vi "Result.vi"(8 "error in (no error)":errorcluster, 10 "Result":T1={"Name"="", "Description"="", "Status"=enum."Passed", "Result Type"=enum."Test Suite", "Execution Time"=0.0, "Data"={"Expected"=variant, "Actual"=variant, "Delta"=variant}}, 11 "Execution Profiler In":refnum<class "Execution Profiler.lvclass">) -> (0 "error out":errorcluster, 3 "Execution Profiler Out":refnum<class "Execution Profiler.lvclass">)   [LabVIEW 2020, in "Execution Profiler.lvclass"]
uses:
  Execution Profiler.lvclass
  Core/Result/Result.ctl
  Core/Result/Status.ctl
  Core/Result/Type.ctl
  Execution Profiler.lvclass/Execution Profiler.ctl
  <vilib>/Utility/miscctls.llb/LVMapReplaceAction.ctl
  Core/Result/Result.lvlib
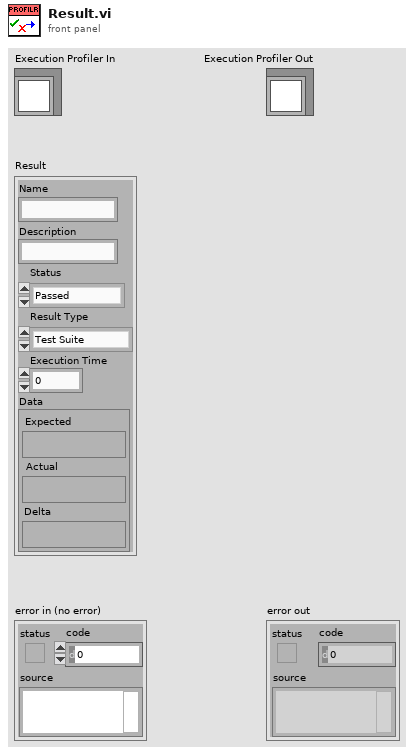
[diagram p1: front panel]
types:
  T1 = typedef "Result.lvlib/Result.ctl" = cluster{"Name":string, "Description":string, "Status":T2, "Result Type":T3, "Execution Time":dbl, "Data":cluster{"Expected":variant, "Actual":variant, "Delta":variant}}
  T2 = typedef "Result.lvlib/Status.ctl" = enum16{"", "Passed", "Failed", "Error", "Skipped", "Setup Error", "Broken", "Teardown Error"}
  T3 = typedef "Result.lvlib/Type.ctl" = enum16{"Test Case", "Test Suite", "Test Run", "Pass", "Fail", "Skip", "Pass if", "Fail if", "Pass if Error", "Fail if Error", "Pass if Equal", "Fail if Equal"}
  T4 = typedef "LVMapReplaceAction.ctl" = enum32{"Modify Entry only if found", "Add or Modify Entry", "Delete Entry"}
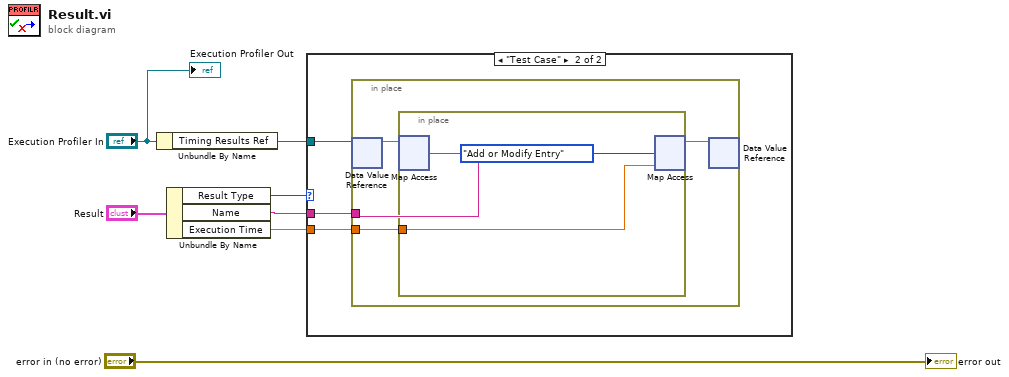
[diagram p0: block diagram]
diagram:
  n1 = Unbundle By Name("Execution Profiler In") -> ("Timing Results Ref"=w5:refnum<data-value>)
  n2 = Unbundle By Name("Result") -> ("Result Type"=w1:T3, "Name"=w4:string, "Execution Time"=w2:dbl)
  n3 = case shown="\"Test Case\"" w1 {
    tunnel: w5 -> [_ w10]
    tunnel: w4 -> [_ w9]
    tunnel: w2 -> [_ w8]
    frame Default {
    }
    frame "Test Case" {
      n4 = in-place {
        in-place-border: w9 -> [w12]
        in-place-border: w8 -> [w11]
        n5 = in-place-dvr #1(w10) -> (w14:map{string, dbl})  [unwired: 1 out]
        n6 = in-place {
          in-place-border: w11 -> [w16]
          n7 = in-place-map #2(w14, w12) -> ()  [unwired: 1 in, 2 out]
          n8 = in-place-map #2(w16, LVMapReplaceAction."Add or Modify Entry" ("action")) -> (w13:map{string, dbl})  [unwired: 2 out]
        }
        n9 = in-place-dvr #1(w13) -> ()  [unwired: 2 out]
      }
    }
  }
  "error out" <- "error in (no error)"
  "Execution Profiler Out" <- "Execution Profiler In"
